vi "Check if Divisible 1-20.vi"(11 "Number to Test?":u64) -> (2 "Passed?":bool, 3 "Number Tested":u64)   [LabVIEW 2013, in "Problem 5.lvlib"]
uses:
  Problem 5.lvlib
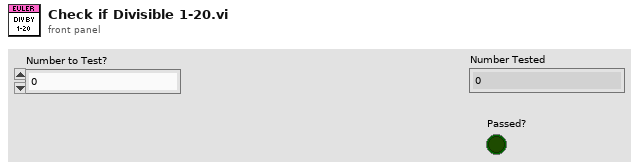
[diagram p1: front panel]
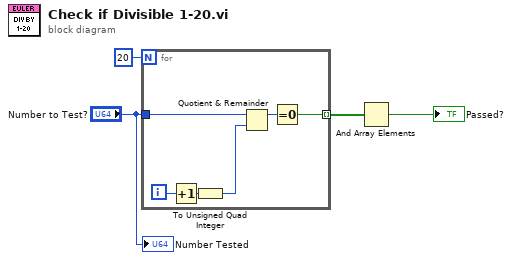
[diagram p0: block diagram]
diagram:
  n1 = for {
    N: 20 -> [_]
    tunnel: "Number to Test?" -> [w9]
    tunnel: [w6] -> w3 mode=indexing
    i -> [w10]
    n2 = Increment(x=w10) -> (x+1=w8:i32)
    n3 = To Unsigned Quad Integer(1:w8) -> (0:w5:u64)
    n4 = Quotient & Remainder(x=w9, y=w5) -> (x-y*floor(x/y)=w7:u64)  [unwired: 1 out]
    n5 = Equal To 0?(x=w7) -> (x = 0?=w6:bool)
  }
  n6 = And Array Elements(Boolean array=w3) -> (logical AND=→"Passed?":bool)
  "Number Tested" <- "Number to Test?"
